vi "Ortalama.vi"() -> ()   [LabVIEW 2015]
uses:
  <vilib>/Analysis/NI_AALBase.lvlib
  <vilib>/Utility/file.llb/Read Delimited Spreadsheet (DBL).vi
  <vilib>/Analysis/baseanly.llb/Mean (DBL).vi
panel:
  out "Veriler":dbl[][](array[numeric])
  in  "Okunacak Veri Adresi":path
  out "Ortalama Hesaplama":dbl
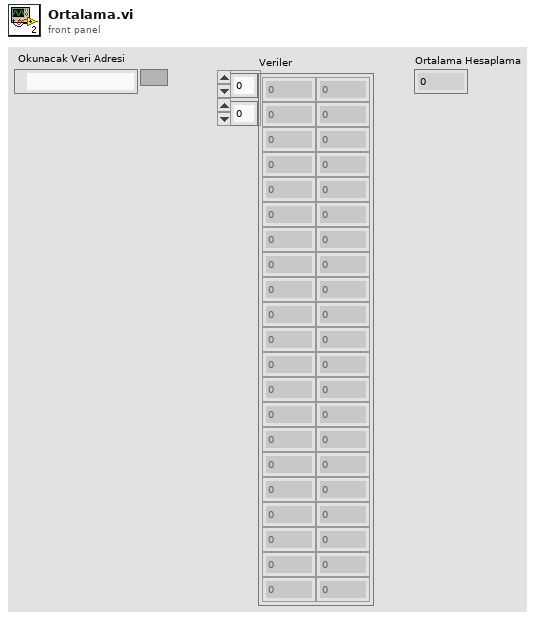
[diagram p1: front panel]
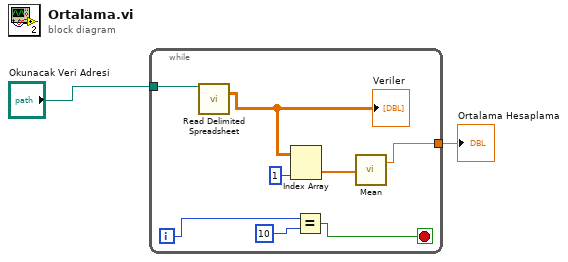
[diagram p0: block diagram]
diagram:
  n1 = while {
    tunnel: "Okunacak Veri Adresi" -> [w10]
    tunnel: [w7] -> w1
    i -> [w6]
    stop <- w4 stop-if-true
    n2 = call-poly <vilib>:"Read Delimited Spreadsheet.vi"("file path (dialog if empty)"=w10) -> ("all rows"=w9:dbl[][])  [unwired: 9 in, 5 out]
    "Veriler" <- w9
    n3 = Index Array(array=w9, index (col)=1 ("disabled index (col)")) -> (element=w8:dbl[])  [unwired: 1 in]
    n4 = Equal?(x=w6, y=10) -> (x = y?=w4:bool)
    n5 = call-poly <vilib>:"Mean.vi"("X"=w8) -> ("mean"=w7:dbl)  [unwired: 1 out]
  }
  "Ortalama Hesaplama" <- w1
